vi "AddMottSchottky.vi"(0 "deviceName":string, 1 "channel":u8, 2 "repeats":u16=1, 3 "startingPotential":sgl, 4 "isStartVoltageVsOCP":bool, 5 "endingPotential":sgl, 6 "isEndVoltageVsOCP":bool, 7 "error in (no error)":errorcluster, 8 "voltageStep":sgl, 9 "startFrequency":sgl, 10 "endFrequency":sgl, 11 "stepsPerDecade":sgl, 12 "amplitude":sgl, 13 "minCycles":u32=2, 14 "quietTime":sgl, 15 "quietTimeSampInterval":sgl=1.0, 16 "stepQuietTime":sgl, 17 "stepQuietSampInterval":sgl=1.0) -> (27 "error out":errorcluster)   [LabVIEW 2018]
doc: "EXPORT void AisAddMottSchottky(const char* deviceName, uint8_t channel, uint16_t repeats, float startingPotential, bool isStartVoltageVsOCP, float endingPotential, bool isEndVoltageVsOCP, float voltageStep, float startFrequency, float endFrequency, float stepsPerDecade, float amplitude, unsigned int minCycles, float quietTime, float quietTimeSampInterval, float stepQuietTime, float stepQuietSampInterval);"
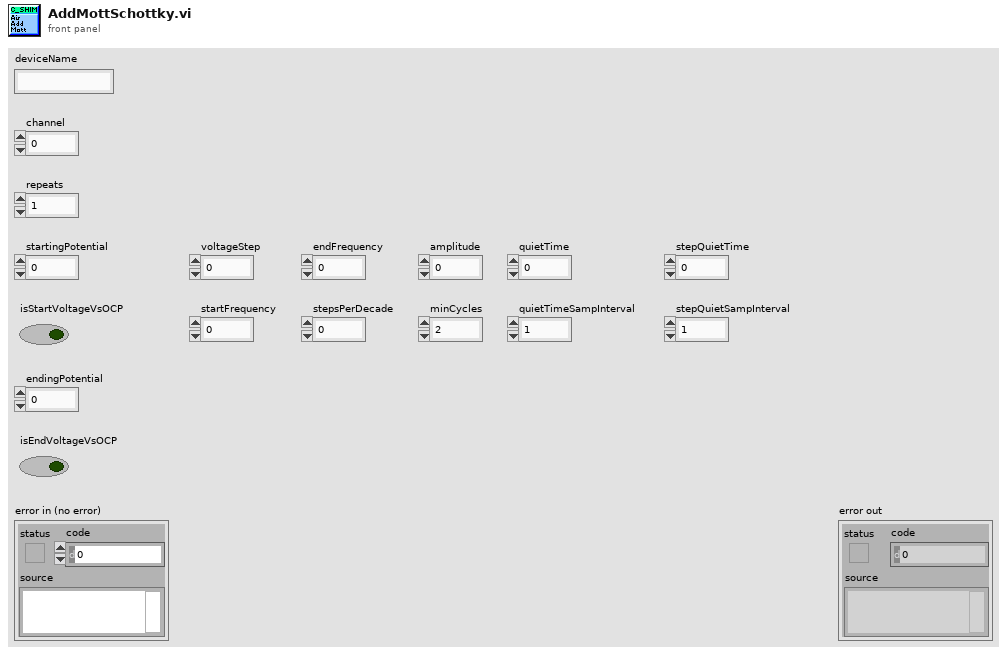
[diagram p1: front panel]
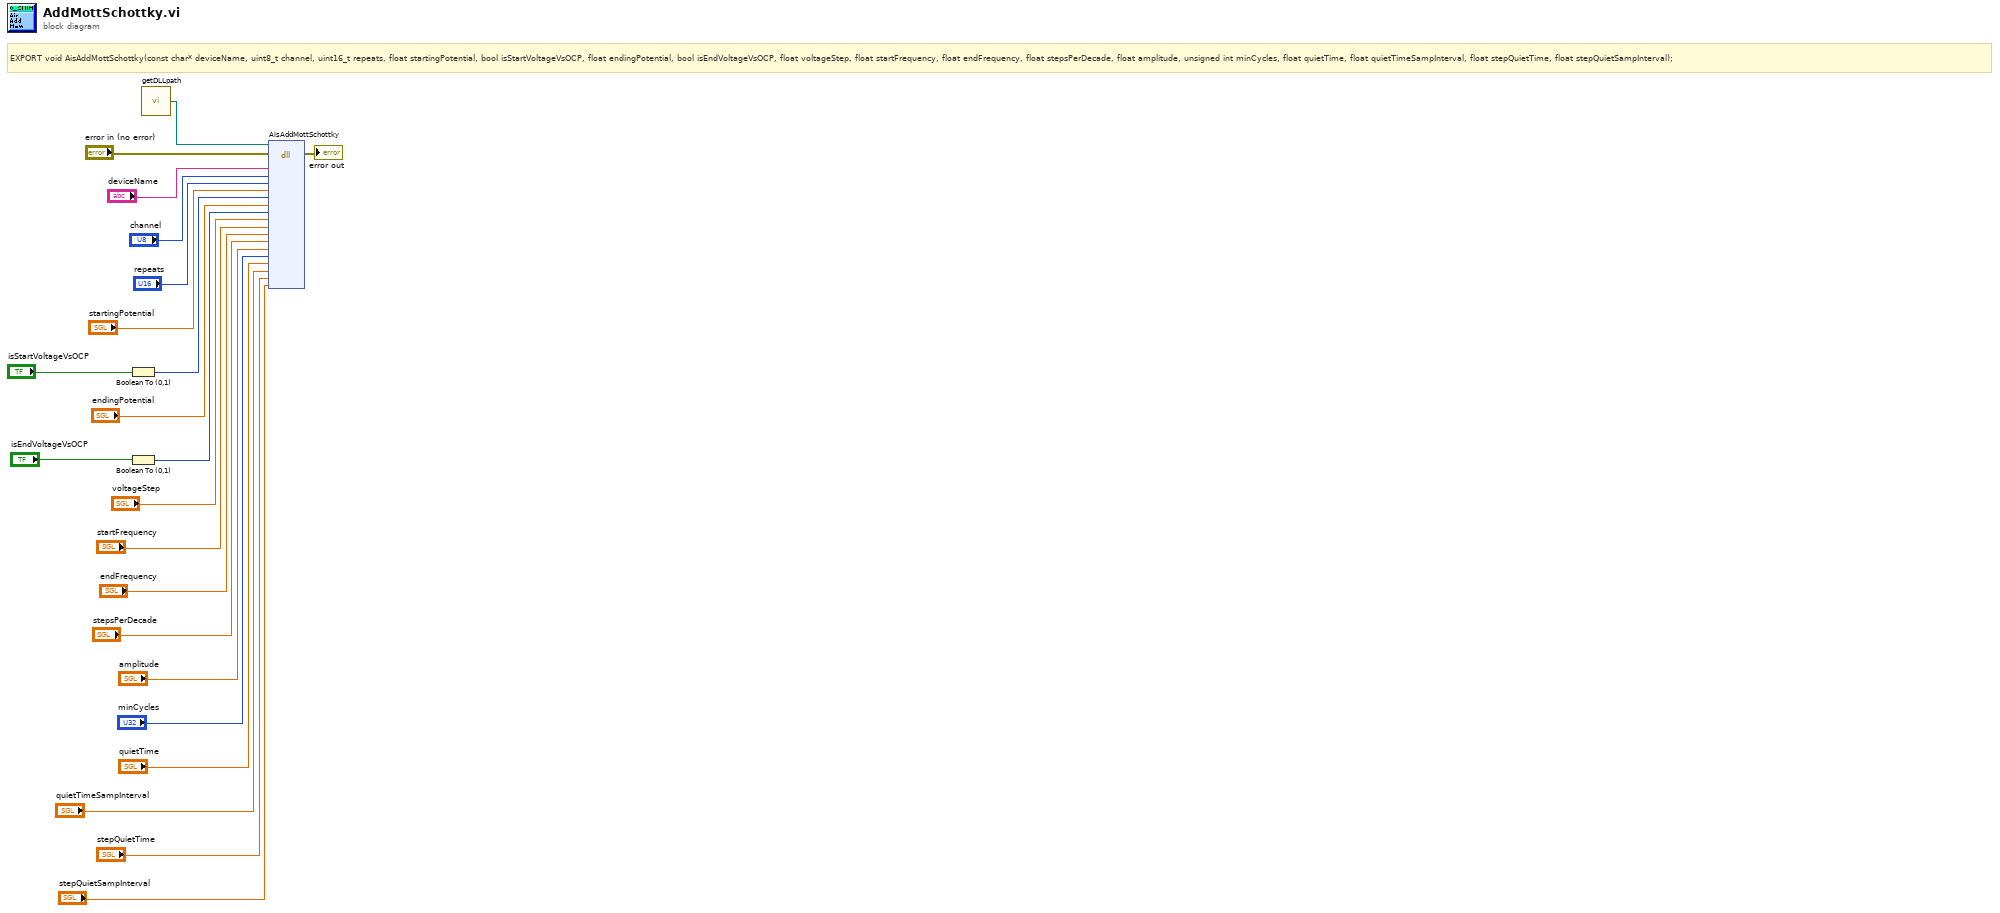
[diagram p0: block diagram]
diagram:
  # "EXPORT void AisAddMottSchottky(const char* deviceName, uint8_t channel, uint16_t repeats, float startingPotential, bool isStartVoltageVsOCP, float endingPotential, bool isEndVoltageVsOCP, float voltageStep, float startFrequency, float endFrequency, float stepsPerDecade, float amplitude, unsigned int minCycles, float quietTime, float quietTimeSampInterval, float stepQuietTime, float stepQuietSampInterval);"
  n1 = Boolean To (0,1)(Boolean="isStartVoltageVsOCP") -> (0, 1=w17:i16)
  n2 = Boolean To (0,1)(Boolean="isEndVoltageVsOCP") -> (0, 1=w14:i16)
  n3 = call "getDLLpath.vi"() -> ("DLL_Path"=w1:path)
  n4 = dll-call lib="?" fn="AisAddMottSchottky"(path in=w1, error in="error in (no error)", "deviceName"="deviceName", "channel"="channel", "repeats"="repeats", "startingPotential"="startingPotential", "isStartVoltageVsOCP"=w17, "endingPotential"="endingPotential", "isEndVoltageVsOCP"=w14, "voltageStep"="voltageStep", "startFrequency"="startFrequency", "endFrequency"="endFrequency", "stepsPerDecade"="stepsPerDecade", "amplitude"="amplitude", "minCycles"="minCycles", "quietTime"="quietTime", "quietTimeSampInterval"="quietTimeSampInterval", "stepQuietTime"="stepQuietTime", "stepQuietSampInterval"="stepQuietSampInterval") -> (error out=→"error out":errorcluster)  [unwired: 19 in, 1 out]
